vi "SineFit.vi"(6 "termination":cluster{"max iteration":i32, "tolerance":dbl}={"max iteration"=2000, "tolerance"=1e-13}, 10 "Frequency":dbl, 11 "Input Data":dbl[](array[numeric])) -> (2 "Phase":dbl, 3 "Amplitude":dbl, 4 "Graph":T1(graph))   [LabVIEW 2015]
uses:
  <vilib>/Analysis/coordinate.llb/Angle Range (Degree).ctl
  <vilib>/Analysis/coordinate.llb/Angle Units.ctl
  <vilib>/Analysis/coordinate.llb/Wrap Angle (scalar).vi
  <vilib>/gmath/NumericalOptimization/Nonlinear Curve Fit LM.vi
  <vilib>/gmath/NI_Gmath.lvlib
  <vilib>/Analysis/NI_AAL_Angle.lvlib
  <vilib>/Analysis/NI_AALPro.lvlib
panel:
  out "Slope":dbl
  in  "X-values":dbl[](array[numeric])
  out "Offset":dbl format="%0.2f"
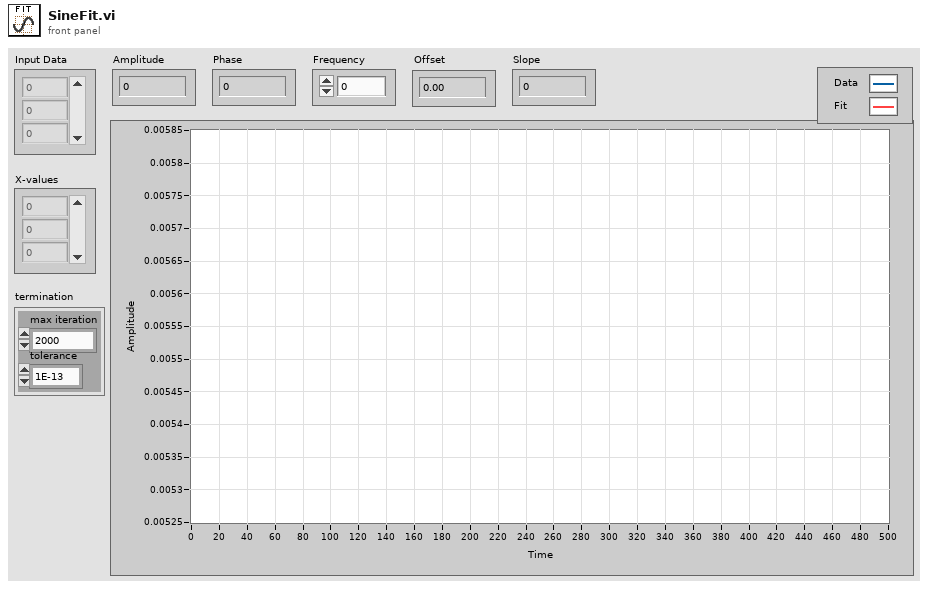
[diagram p1: front panel]
types:
  T1 = cluster{"X-values":dbl[], "best nonlinear fit":dbl[]}[]
  T2 = typedef "NI_AAL_Angle.lvlib/Angle Units.ctl" = i32
  T3 = typedef "NI_AAL_Angle.lvlib/Angle Range (Degree).ctl" = u16
  T4 = cluster{"X-values":dbl[], "best nonlinear fit":dbl[]}
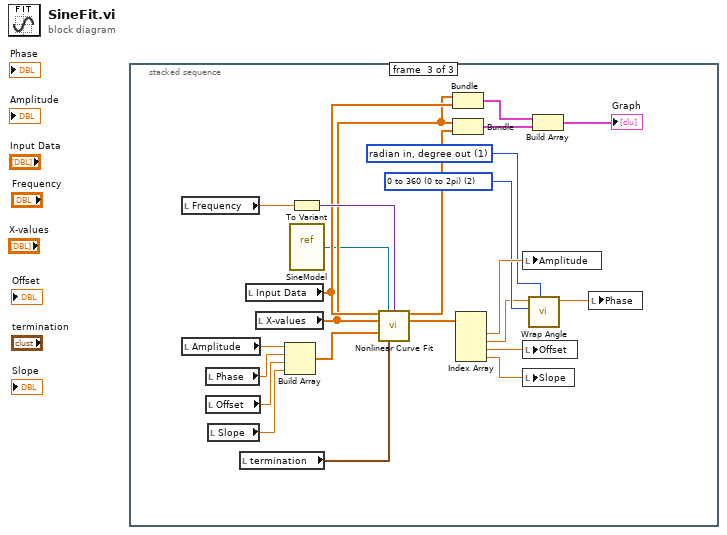
[diagram p0: block diagram]
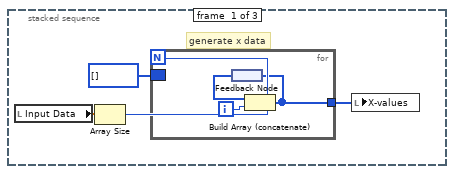
[diagram p2: hidden frame]
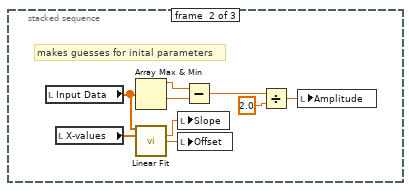
[diagram p3: hidden frame]
diagram:
  n1 = stacked-sequence {
    frame #0 {
      # "generate x data"
      n2 = local read "Input Data"() -> (w2:dbl[])
      n3 = Array Size(array=w2) -> (size(s)=w4:i32)
      n4 = for {
        N: w4 -> [_]
        border: i32[] [] -> [_]
        tunnel: [w5] -> w1
        i -> [w6]
        n5 = feedback #1() -> (w7:i32[])
        n6 = Build Array (concatenate)(w7, w6) -> (w5:i32[])
        n7 = feedback-in #1(w5) -> ()
      }
      n8 = local write "X-values"(w1) -> ()
    }
    frame #1 {
      # "makes guesses for inital parameters"
      n9 = local read "Input Data"() -> (w10:dbl[])
      n10 = local read "X-values"() -> (w11:dbl[])
      n11 = Array Max & Min(array=w10) -> (max value=w15:dbl, min value=w16:dbl)  [unwired: 2 out]
      n12 = call <vilib>:"Linear Fit.vi"("Y"=w10, "X"=w11) -> ("slope"=w9:dbl, "intercept"=w8:dbl)  [unwired: 9 in, 3 out]
      n13 = local write "Slope"(w9) -> ()
      n14 = local write "Offset"(w8) -> ()
      n15 = Subtract(x=w15, y=w16) -> (x-y=w14:dbl)
      n16 = Divide(x=w14, y=2.0) -> (x/y=w12:dbl)
      n17 = local write "Amplitude"(w12) -> ()
    }
    frame #2 {
      w23 = T2 1 items=["radian in, radian out", "radian in, degree out", "degree in, degree out", "degree in, radian out"] ("angle units")
      w24 = T3 2 items=["none", "-180 to 180 (-pi to pi)", "0 to 360 (0 to 2pi)"] ("angle range")
      n18 = local read "Frequency"() -> (w35:dbl)
      n19 = local read "Amplitude"() -> (w39:dbl)
      n20 = local read "Phase"() -> (w38:dbl)
      n21 = local read "Offset"() -> (w37:dbl)
      n22 = local read "Slope"() -> (w18:dbl)
      n23 = local read "termination"() -> (w19:cluster{"max iteration":i32, "tolerance":dbl})
      n24 = local read "Input Data"() -> (w26:dbl[])
      n25 = local read "X-values"() -> (w25:dbl[])
      n26 = Build Array(w39, w38, w37, w18) -> (w36:dbl[])
      n27 = vi-ref "SineModel.vi"() -> (w21:refnum<vi>)
      n28 = To Variant(anything=w35) -> (Variant=w34:variant)
      n29 = call-poly <vilib>:"Nonlinear Curve Fit.vi"("Y"=w26, "f(x,a)"=w21, "data"=w34, "X"=w25, "initial parameters"=w36, "termination"=w19) -> ("best nonlinear fit"=w30:dbl[], "best fit parameters"=w33:dbl[])  [unwired: 4 in, 4 out]
      n30 = Bundle("X-values"=w25, "Input Data"=w26) -> (w29:cluster{"X-values":dbl[], "Input Data":dbl[]})  [unwired: 1 in]
      n31 = Bundle("X-values"=w25, "best nonlinear fit"=w30) -> (w28:T4)  [unwired: 1 in]
      n32 = Index Array(array=w33) -> (element #1=w32:dbl, element #2=w22:dbl, element #3=w31:dbl, element #4=w17:dbl)  [unwired: 4 in]
      n33 = local write "Amplitude"(w32) -> ()
      n34 = local write "Offset"(w31) -> ()
      n35 = local write "Slope"(w17) -> ()
      n36 = call-poly <vilib>:"Wrap Angle.vi"("angle units"=w23, "angle range"=w24, "angle in"=w22) -> ("angle out"=w20:dbl)  [unwired: 7 in, 1 out]
      n37 = Build Array(w29, w28) -> (→"Graph":T1)
      n38 = local write "Phase"(w20) -> ()
    }
  }
